vi "neuron-mcu.vi"(8 "Weights":i32[](array[numeric]), 11 "Inputs":i32[](array[numeric])) -> (0 "Error?":bool, 3 "Output":dbl)   [LabVIEW 2015]
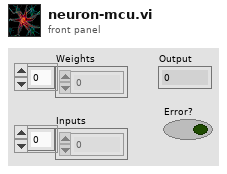
[diagram p1: front panel]
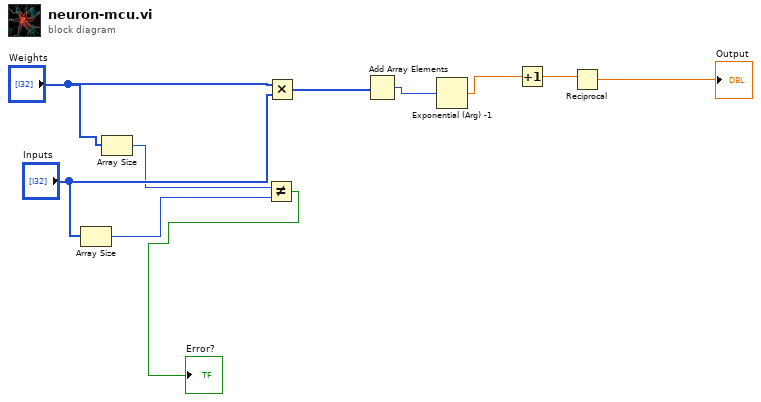
[diagram p0: block diagram]
diagram:
  n1 = Array Size(array="Inputs") -> (size(s)=w10:i32)
  n2 = Array Size(array="Weights") -> (size(s)=w8:i32)
  n3 = Not Equal?(x=w8, y=w10) -> (x != y?=→"Error?":bool)
  n4 = Multiply(x="Weights", y="Inputs") -> (x*y=w1:i32[])
  n5 = Add Array Elements(numeric array=w1) -> (sum=w2:i32)
  n6 = Exponential (Arg) -1(1:w2) -> (0:w3:dbl)
  n7 = Increment(x=w3) -> (x+1=w4:dbl)
  n8 = Reciprocal(x=w4) -> (1/x=→"Output":dbl)
